vi "VIP_Pre-Uninstall Custom Action.vi"(10 "Variant":variant) -> (0 "error out":errorcluster)   [LabVIEW 2021]
uses:
  <vilib>/regexp/Match Regular Expression.xnode
  <vilib>/Utility/sysdir.llb/System Directory Type.ctl
  <userlib>/_OpenG.lib/file/file.llb/openg_file.lvlib
  <userlib>/_OpenG.lib/file/file.llb/Build Path - Traditional__ogtk.vi
  <userlib>/_OpenG.lib/lvzip/lvzip.llb/subVI/ZLIB Extract All Files To Dir (Path)__ogtk.vi
  <resource>/dialog/lvconfig.llb/LV Config Read String.vi
panel:
  # "pre uninstall"
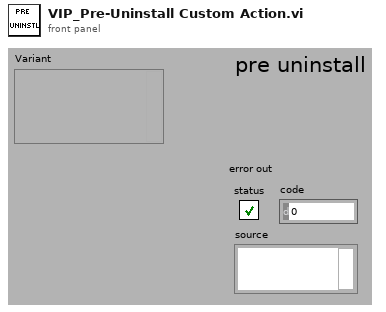
[diagram p1: front panel]
types:
  T1 = typedef "System Directory Type.ctl" = i32
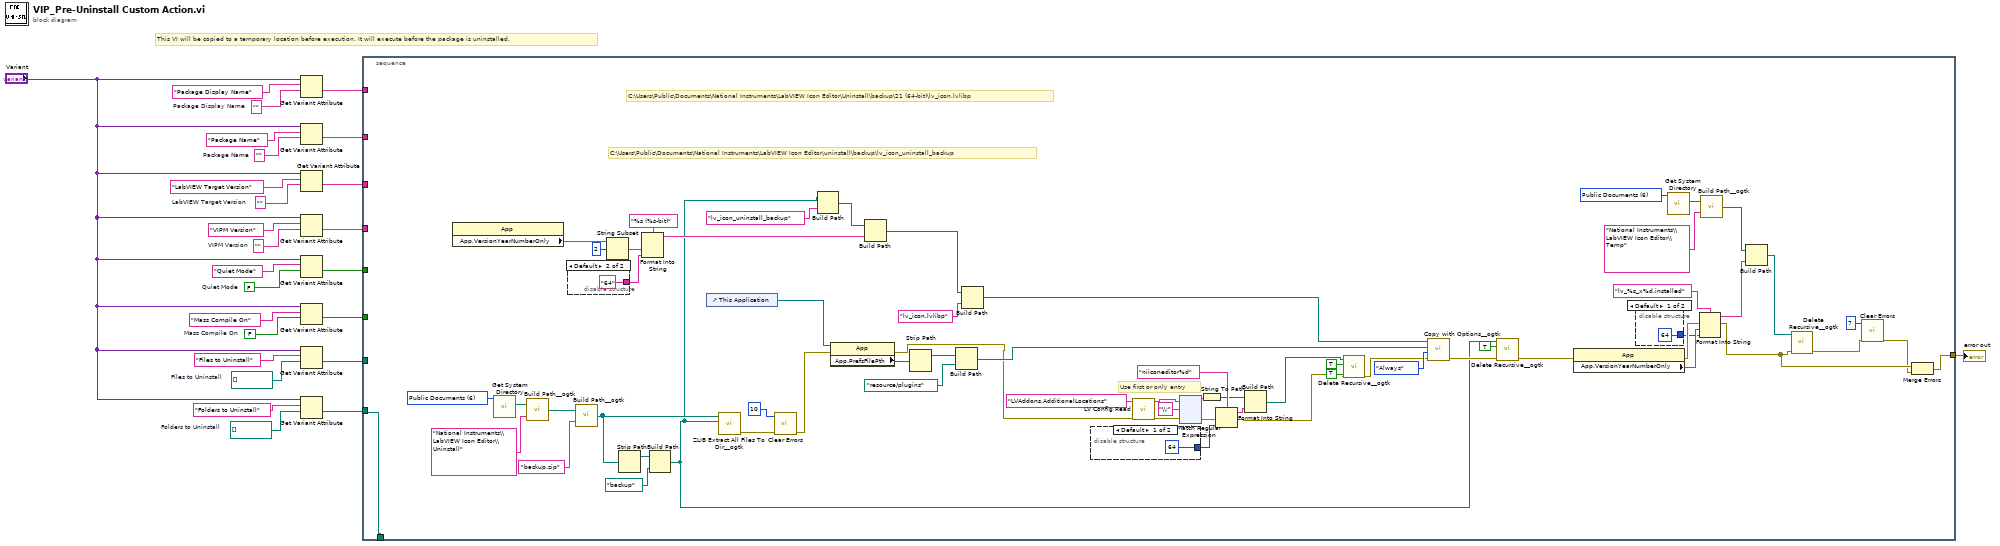
[diagram p0: block diagram]
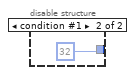
[diagram p2: hidden frame]
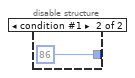
[diagram p3: hidden frame]
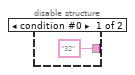
[diagram p4: hidden frame]
diagram:
  w11 = path[] []  # Folders to Uninstall
  w14 = path[] []  # Files to Uninstall
  w15 = FALSE  # Mass Compile On
  w16 = ""  # Package Display Name
  w17 = FALSE  # Quiet Mode
  w20 = ""  # VIPM Version
  w22 = ""  # LabVIEW Target Version
  w24 = ""  # Package Name
  # "This VI will be copied to a temporary location before execution. It will execute before the package is uninstalled."
  n1 = Get Variant Attribute(Variant="Variant", name="Package Display Name", default value (empty Variant)=w16) -> (value=w9:string)  [unwired: 1 in, 3 out]
  n2 = Get Variant Attribute(Variant="Variant", name="Package Name", default value (empty Variant)=w24) -> (value=w8:string)  [unwired: 1 in, 3 out]
  n3 = Get Variant Attribute(Variant="Variant", name="LabVIEW Target Version", default value (empty Variant)=w22) -> (value=w7:string)  [unwired: 1 in, 3 out]
  n4 = Get Variant Attribute(Variant="Variant", name="VIPM Version", default value (empty Variant)=w20) -> (value=w6:string)  [unwired: 1 in, 3 out]
  n5 = Get Variant Attribute(Variant="Variant", name="Quiet Mode", default value (empty Variant)=w17) -> (value=w5:bool)  [unwired: 1 in, 3 out]
  n6 = Get Variant Attribute(Variant="Variant", name="Mass Compile On", default value (empty Variant)=w15) -> (value=w4:bool)  [unwired: 1 in, 3 out]
  n7 = Get Variant Attribute(Variant="Variant", name="Folders to Uninstall", default value (empty Variant)=w11) -> (value=w2:path[])  [unwired: 1 in, 3 out]
  n8 = Get Variant Attribute(Variant="Variant", name="Files to Uninstall", default value (empty Variant)=w14) -> (value=w3:path[])  [unwired: 1 in, 3 out]
  n9 = stacked-sequence {
    tunnel: w9 -> [_]
    tunnel: w8 -> [_]
    tunnel: w7 -> [_]
    tunnel: w6 -> [_]
    tunnel: w5 -> [_]
    tunnel: w4 -> [_]
    tunnel: w3 -> [_]
    tunnel: w2 -> [w27]
    tunnel: [w44] -> w1
    tunnel: [w27] -> _
    frame #0 {
      w60 = T1 6 items=["User Home"=0, "User Desktop"=1, "User Documents"=2, "User Application Data"=3, "User Preferences"=4, "User Temporary"=5, "Public Documents"=6, "Public Application Data"=7, "Public Preferences"=8, "Public Cache"=13, "System Core Libraries"=9, "System Installed Libraries"=10, "Application Files"=11, "Boot Volume Root"=12] ("system directory type")
      w75 = T1 6 items=["User Home"=0, "User Desktop"=1, "User Documents"=2, "User Application Data"=3, "User Preferences"=4, "User Temporary"=5, "Public Documents"=6, "Public Application Data"=7, "Public Preferences"=8, "Public Cache"=13, "System Core Libraries"=9, "System Installed Libraries"=10, "Application Files"=11, "Boot Volume Root"=12] ("system directory type")
      # "Use first or only entry"
      # "C:\\Users\\Public\\Documents\\National Instruments\\LabVIEW Icon Editor\\uninstall\\backup\\lv_icon_uninstall_backup"
      # "C:\\Users\\Public\\Documents\\National Instruments\\LabVIEW Icon Editor\\Uninstall\\backup\\21 (64-bit)\\lv_icon.lvlibp"
      n10 = property class="App"() -> ("App.VersionYearNumberOnly"=w79:string)  [unwired: 2 in, 2 out]
      n11 = call <vilib>:"Get System Directory.vi"("system directory type"=w75) -> ("system directory"=w74:path)  [unwired: 10 in]
      n12 = call-poly <userlib>:"Build Path__ogtk.vi"("name or relative path"="National Instruments\\LabVIEW Icon Editor\\Uninstall", "base path"=w74) -> ("appended path"=w71:path)
      n13 = disable-structure shown="Default" {
        disable-tunnel: ["32" "64"] -> w89
        frame condition #0 {
        }
        frame condition #1 (active) {
        }
      }
      n14 = call-poly <userlib>:"Build Path__ogtk.vi"("name or relative path"="backup.zip", "base path"=w71) -> ("appended path"=w66:path)
      n15 = String Subset(string=w79, offset (0)=2) -> (substring=w78:string)  [unwired: 1 in]
      n16 = Strip Path(path=w66) -> (stripped path=w70:path)  [unwired: 1 out]
      n17 = Format Into String(format string="%s (%s-bit)", w78, w89) -> (resulting string=w82:string)  [unwired: 2 in, 1 out]
      n18 = Build Path(base path=w70, name or relative path=path "backup") -> (appended path=w52:path)
      n19 = control-ref of="This Application"() -> (w76:refnum<vi>)
      n20 = call-poly <userlib>:"ZLIB Extract All Files To Dir__ogtk.vi"("destination directory (archive name without ending)"=w52, "archive name (file dialog)"=w66) -> ("error out"=w55:errorcluster)  [unwired: 7 in, 2 out]
      n21 = call <vilib>:"Clear Errors.vi"("error in (no error)"=w55, "specific error code to clear (0: all)"=10) -> ("error out"=w54:errorcluster)  [unwired: 4 in, 1 out]
      n22 = Build Path(base path=w52, name or relative path="lv_icon_uninstall_backup" ("resulting string")) -> (appended path=w51:path)
      n23 = property class="App"(reference=w76, error in=w54) -> (error out=w81:errorcluster, "App.PrefsFilePth"=w88:path)  [unwired: 1 out]
      n24 = Build Path(base path=w51, name or relative path=w82) -> (appended path=w77:path)
      n25 = Strip Path(path=w88) -> (stripped path=w87:path)  [unwired: 1 out]
      n26 = Build Path(base path=w87, name or relative path=path "resource/plugins") -> (appended path=w85:path)
      n27 = Build Path(base path=w77, name or relative path="lv_icon.lvlibp" ("resulting string")) -> (appended path=w83:path)
      n28 = disable-structure shown="Default" {
        disable-tunnel: [64 ("code") 32 ("code")] -> w37
        frame condition #0 (active) {
        }
        frame condition #1 {
        }
      }
      n29 = call-poly <resource>:"LV Config Read.vi"("error in"=w81, "key"="LVAddons.AdditionalLocations") -> ("error out"=w38:errorcluster, "value"=w36:string)  [unwired: 3 in, 1 out]
      n30 = xnode "Match Regular Expression"("input string"=w36, "regular expression"="\\;", "error in"=w38) -> ("before match"=w31:string, "error out"=w39:errorcluster)  [unwired: 3 in, 3 out]
      n31 = String To Path(string=w31) -> (path=w30:path)
      n32 = Format Into String(format string="niiconeditor%d", error in=w39, w37) -> (resulting string=w29:string, error out=w32:errorcluster)  [unwired: 1 in]
      n33 = Build Path(base path=w30, name or relative path=w29) -> (appended path=w28:path)
      n34 = call <userlib>:"Delete Recursive__ogtk.vi"("error in (no error)"=w32, "Ignore Read-Only? (FALSE)"=TRUE, "Recursive? (FALSE)"=TRUE, "Path"=w28) -> ("error out"=w42:errorcluster)  [unwired: 6 in, 1 out]
      n35 = call <userlib>:"Copy with Options__ogtk.vi"("error in (no error)"=w42, "Replace Mode (Never)"=enum16{"Never", "Always", "If Newer"}."Always", "target path"=w85, "source path"=w83) -> ("error out"=w65:errorcluster)  [unwired: 6 in, 1 out]
      n36 = call <userlib>:"Delete Recursive__ogtk.vi"("error in (no error)"=w65, "Recursive? (FALSE)"=TRUE, "Path"=w52) -> ("error out"=w64:errorcluster)  [unwired: 7 in, 1 out]
      n37 = property class="App"(error in=w64) -> (error out=w67:errorcluster, "App.VersionYearNumberOnly"=w59:string)  [unwired: 1 in, 1 out]
      n38 = disable-structure shown="Default" {
        disable-tunnel: [64 ("code") 86 ("code")] -> w58
        frame condition #0 (active) {
        }
        frame condition #1 {
        }
      }
      n39 = call <vilib>:"Get System Directory.vi"("system directory type"=w60) -> ("system directory"=w61:path)  [unwired: 10 in]
      n40 = Format Into String(format string="lv_%s_x%d.installed", error in=w67, w59, w58) -> (resulting string=w57:string, error out=w46:errorcluster)  [unwired: 1 in]
      n41 = call-poly <userlib>:"Build Path__ogtk.vi"("name or relative path"="National Instruments\\LabVIEW Icon Editor\\Temp", "base path"=w61) -> ("appended path"=w56:path)
      n42 = Build Path(base path=w56, name or relative path=w57) -> (appended path=w49:path)
      n43 = call <userlib>:"Delete Recursive__ogtk.vi"("error in (no error)"=w46, "Path"=w49) -> ("error out"=w48:errorcluster)  [unwired: 8 in, 1 out]
      n44 = call <vilib>:"Clear Errors.vi"("error in (no error)"=w48, "specific error code to clear (0: all)"=7) -> ("error out"=w45:errorcluster)  [unwired: 4 in, 1 out]
      n45 = Merge Errors(w46, w45) -> (w44:errorcluster)
    }
  }
  "error out" <- w1
